vi "Analysis.Result Summaries, TE History, Generate Pareto.vi"(11 "Test History":T1) -> (0 "Test Time Histogram":T4(graph), 1 "Test Times (s)":cluster{"Min":dbl, "Max":dbl, "Avg":dbl}, 2 "Metrics":T5 {"Yield%" format="%.2f"}, 3 "FP Pareto":string[][](table))   [LabVIEW 2024]
uses:
  Analysis.Result Summary, Metrics.ctl
  TestExec/TestExec.Test Result Metric History.ctl
  TestExec/TestExec.Test Result Metric History Item.ctl
  <vilib>/KATE/SeqMgr/SeqMgr.Result State Enum.ctl
  <vilib>/Analysis/NI_AALBase.lvlib
  <vilib>/KATE/SeqMgr/SeqMgr.lvlib
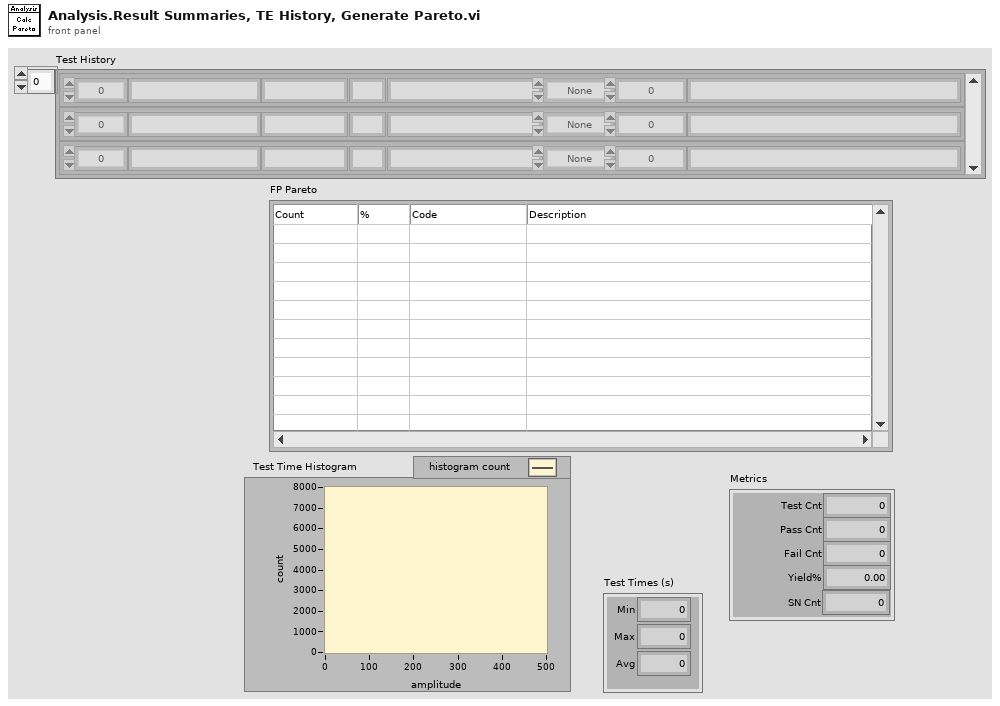
[diagram p1: front panel]
types:
  T1 = typedef "TestExec.Test Result Metric History.ctl" = T2[]
  T2 = typedef "TestExec.Test Result Metric History Item.ctl" = cluster{"TimeStamp":timestamp, "Dur(s)":dbl, "Time":string, "Mode ":string, "Test ":string, "SN":string, "State":T3, "Code":i32, "Description":string, "Pos ":string}
  T3 = typedef "KATE_Lib.lvlib/SeqMgr.lvlib/SeqMgr.Result State Enum.ctl" = enum16{"None", "Passing", "Failing", "PASS", "FAIL", "ABORT", "ERROR"}
  T4 = cluster{"X Values":dbl[], "Histogram: h(x)":i32[]}
  T5 = typedef "Analysis.Result Summary, Metrics.ctl" = cluster{"Pass Cnt":i32, "Fail Cnt":i32, "Yield%":dbl, "Test Cnt":i32, "SN Cnt":i32}
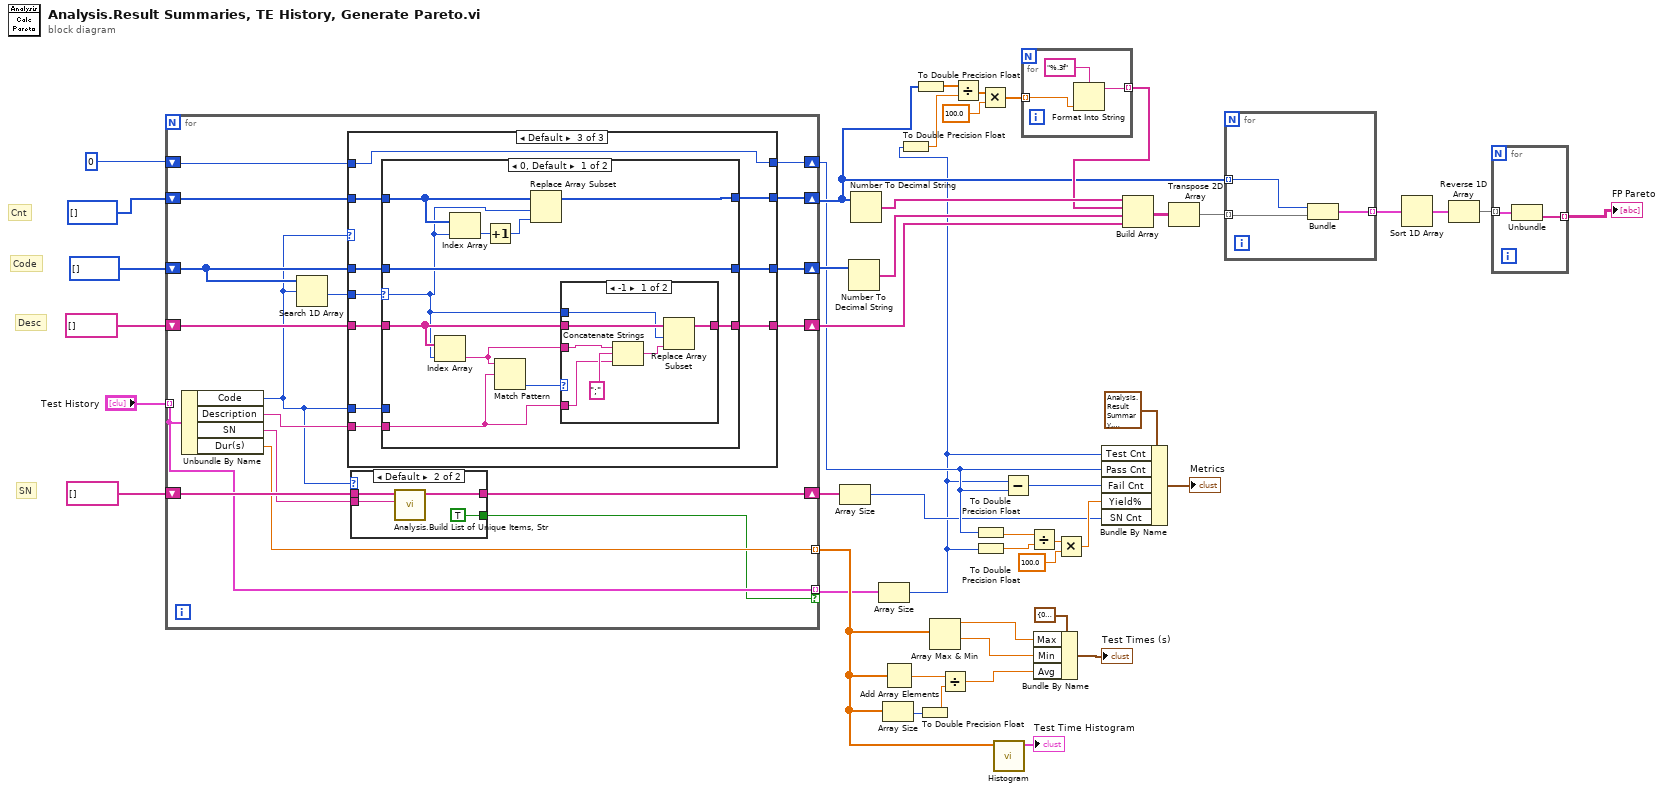
[diagram p0: block diagram]
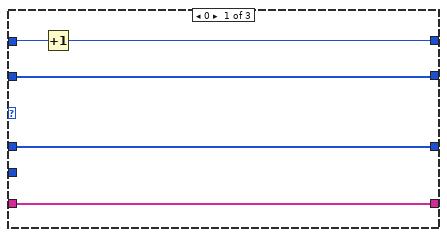
[diagram p3: hidden frame]
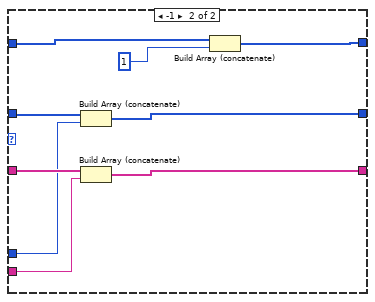
[diagram p6: hidden frame]
diagram:
  # "SN"
  # "Desc"
  # "Code"
  # "Cnt"
  n1 = for {
    shift-right: [w59] -> w30
    shift-left: i32[] [] -> [w62]
    shift-right: [w58] -> w27
    shift-left: i32[] [] -> [w61]
    shift-right: [w57] -> w43
    shift-left: string[] [] -> [w60]
    tunnel: "Test History" -> [w48] mode=indexing
    shift-right: [w55] -> w17
    shift-left: 0 ("Numeric") -> [w56]
    shift-right: [w51] -> w24
    shift-left: string[] [] -> [w53]
    tunnel: [w50] -> w11 mode=indexing
    tunnel: [w48] -> w2 mode=indexing if=w47
    n2 = Unbundle By Name(w48) -> ("Code"=w49:i32, "Description"=w54:string, "SN"=w52:string, "Dur(s)"=w50:dbl)
    n3 = Search 1D Array(1D array=w61, element=w49) -> (index of element=w63:i32)  [unwired: 1 in]
    n4 = case shown="Default" w49 {
      tunnel: w63 -> [_ _ w87]
      tunnel: w62 -> [w73 w76 w86]
      tunnel: w61 -> [w72 w75 w85]
      tunnel: w60 -> [w71 w74 w84]
      tunnel: [w73 w76 w83] -> w59
      tunnel: [w72 w75 w82] -> w58
      tunnel: [w71 w74 w81] -> w57
      tunnel: w49 -> [_ _ w80]
      tunnel: w54 -> [_ _ w79]
      tunnel: w56 -> [w70 w77 w78]
      tunnel: [w69 w77 w78] -> w55
      frame 0 {
        n5 = Increment(x=w70) -> (x+1=w69:i32)
      }
      frame -1 {
        # "Ignore aborts"
      }
      frame Default {
        n6 = case shown="0, Default" w87 {
          selector: w87 -> [w88 _]
          tunnel: w86 -> [w97 w112]
          tunnel: w85 -> [w94 w114]
          tunnel: w84 -> [w92 w115]
          tunnel: [w98 w111] -> w83
          tunnel: [w94 w110] -> w82
          tunnel: [w91 w109] -> w81
          tunnel: w80 -> [_ w107]
          tunnel: w79 -> [w89 w108]
          frame 0, Default {
            n7 = Index Array(array=w92, index=w88) -> (element=w90:string)
            n8 = Index Array(array=w97, index=w88) -> (element=w96:i32)
            n9 = Increment(x=w96) -> (x+1=w95:i32)
            n10 = Match Pattern(string=w90, regular expression=w89) -> (offset past match=w93:i32)  [unwired: 1 in, 3 out]
            n11 = Replace Array Subset(array=w97, new element=w95, index=w88) -> (w98:i32[])
            n12 = case shown="-1" w93 {
              tunnel: w92 -> [w104 w106]
              tunnel: [w105 w106] -> w91
              tunnel: w90 -> [w103 _]
              tunnel: w89 -> [w101 _]
              tunnel: w88 -> [w99 _]
              frame -1 {
                n13 = Concatenate Strings(w103, ";", w101) -> (w100:string)
                n14 = Replace Array Subset(array=w104, new element=w100, index=w99) -> (w105:string[])
              }
              frame Default {
              }
            }
          }
          frame -1 {
            n15 = Build Array (concatenate)(w114, w107) -> (w110:i32[])
            n16 = Build Array (concatenate)(w115, w108) -> (w109:string[])
            n17 = Build Array (concatenate)(w112, 1) -> (w111:i32[])
          }
        }
      }
    }
    n18 = case shown="Default" w49 {
      tunnel: w53 -> [w64 w68]
      tunnel: w52 -> [_ w67]
      tunnel: [w64 w66] -> w51
      tunnel: [_ TRUE] -> w47
      frame -1 {
      }
      frame Default {
        n19 = call "Analysis.Build List of Unique Items, Str.vi"("Item In"=w67, "List In"=w68) -> ("List Out"=w66:string[])  [unwired: 7 in, 2 out]
      }
    }
  }
  n20 = Array Size(array=w24) -> (size(s)=w4:i32)
  n21 = Number To Decimal String(number=w27) -> (decimal integer string=w26:string[])  [unwired: 1 in]
  n22 = Number To Decimal String(number=w30) -> (decimal integer string=w32:string[])  [unwired: 1 in]
  n23 = Array Size(array=w2) -> (size(s)=w1:i32)
  n24 = Array Size(array=w11) -> (size(s)=w12:i32)
  n25 = Add Array Elements(numeric array=w11) -> (sum=w14:dbl)
  n26 = To Double Precision Float(number=w1) -> (double precision float=w28:dbl)
  n27 = To Double Precision Float(number=w30) -> (double precision float=w29:dbl[])
  n28 = To Double Precision Float(number=w12) -> (double precision float=w13:dbl)
  n29 = Array Max & Min(array=w11) -> (max value=w5:dbl, min value=w6:dbl)  [unwired: 2 out]
  n30 = Divide(x=w14, y=w13) -> (x/y=w7:dbl)
  n31 = Divide(x=w29, y=w28) -> (x/y=w33:dbl[])
  n32 = To Double Precision Float(number=w17) -> (double precision float=w20:dbl)
  n33 = To Double Precision Float(number=w1) -> (double precision float=w21:dbl)
  n34 = Multiply(x=w33, y=100.0) -> (x*y=w35:dbl[])
  n35 = call <vilib>:"Histogram.vi"("X"=w11) -> ("Histogram Graph"=→"Test Time Histogram":T4)  [unwired: 7 in, 3 out]
  n36 = Subtract(x=w1, y=w17) -> (x-y=w22:i32)
  n37 = for {
    tunnel: w35 -> [w117] mode=indexing
    tunnel: [w116] -> w31 mode=indexing
    n38 = Format Into String(format string="%.3f", w117) -> (resulting string=w116:string)  [unwired: 2 in, 1 out]
  }
  n39 = Divide(x=w20, y=w21) -> (x/y=w19:dbl)
  n40 = Bundle By Name(cluster=cluster{"Min":dbl, "Max":dbl, "Avg":dbl} {"Min"=0.0, "Max"=0.0, "Avg"=0.0} ("Test Times (s)"), "Max"=w5, "Min"=w6, "Avg"=w7) -> (→"Test Times (s)":cluster{"Min":dbl, "Max":dbl, "Avg":dbl})
  n41 = Multiply(x=w19, y=100.0) -> (x*y=w16:dbl)
  n42 = Bundle By Name(cluster=T5 {"Pass Cnt"=5050, "Fail Cnt"=374, "Yield%"=93.1047197640118, "Test Cnt"=5424, "SN Cnt"=374} ("Metrics"), "Test Cnt"=w1, "Pass Cnt"=w17, "Fail Cnt"=w22, "Yield%"=w16, "SN Cnt"=w4) -> (→"Metrics":T5)
  n43 = Build Array(w32, w31, w26, w43) -> (w42:string[][])
  n44 = Transpose 2D Array(2D array=w42) -> (transposed array=w41:string[][])
  n45 = for {
    tunnel: w41 -> [w119] mode=indexing
    tunnel: w30 -> [w121] mode=indexing
    tunnel: [w120] -> w39 mode=indexing
    n46 = Bundle("Numeric"=w121, w119) -> (w120:cluster{"Numeric":i32, string[]})  [unwired: 1 in]
  }
  n47 = Sort 1D Array(array=w39) -> (sorted array=w38:cluster{"Numeric":i32, string[]}[])
  n48 = Reverse 1D Array(array=w38) -> (reversed array=w37:cluster{"Numeric":i32, string[]}[])
  n49 = for {
    tunnel: w37 -> [w123] mode=indexing
    tunnel: [w122] -> w36 mode=indexing
    n50 = Unbundle(w123) -> (w122:string[])  [unwired: 1 out]
  }
  "FP Pareto" <- w36
